vi "Get Key Line.vi"(10 "key description":string, 11 "info data":string) -> (3 "key value":string)   [LabVIEW 2019, in "infolib.lvlib"]
doc: "Remove all sections and returns the rest. Contain infinite loop, but every iteration something should be removed, so the loop should always end."
uses:
  infolib.lvlib
  <vilib>/regexp/Match Regular Expression.xnode
panel:
  # "testing string:"
  # "test1 :: 1\ntest2 :: 22\n#startsection:: 1\nAAA\n#startsection:: 2\nBBB\n\t  \t#endsection:: 2\nCCC\n#endsection:: 1\ntest3::333\n   test4:: 4444\n#startsection:: X\nDDD\n#endsection:: X\ntest5"
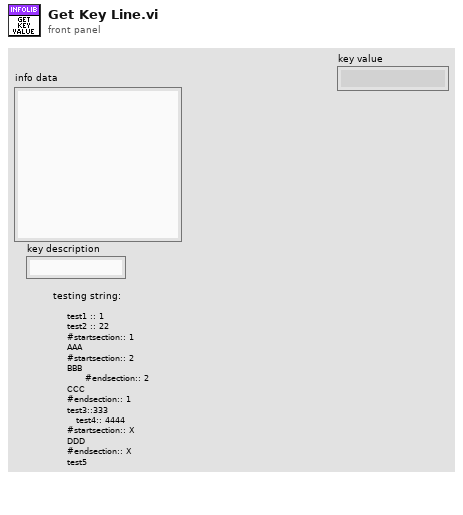
[diagram p1: front panel]
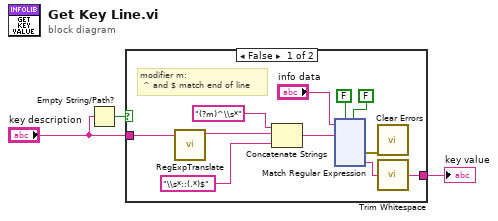
[diagram p0: block diagram]
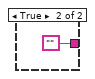
[diagram p2: hidden frame]
diagram:
  n1 = Empty String/Path?(string/path="key description") -> (empty?=w1:bool)
  n2 = case shown="False" w1 {
    tunnel: [w8 ""] -> w3
    tunnel: "key description" -> [w7 _]
    frame False {
      # "modifier m:\n ^ and $ match end of line"
      n3 = call "RegExpTranslate.vi"("string"=w7) -> ("regexp safe string"=w6:string)  [unwired: 10 in]
      n4 = Concatenate Strings("(?m)^\\s*" ("section name"), w6, "\\s*::(.*)$" ("section name")) -> (w9:string)
      n5 = xnode "Match Regular Expression"("input string"="info data", "regular expression"=w9, "ignore case? (F)"=FALSE, "multiline? (F)"=FALSE) -> ("error out"=w13:errorcluster, "submatch 1"=w12:string)  [unwired: 2 in, 4 out]
      n6 = call <vilib>:"Clear Errors.vi"("error in (no error)"=w13) -> ()  [unwired: 5 in, 2 out]
      n7 = call <vilib>:"Trim Whitespace.vi"("string"=w12) -> ("trimmed string"=w8:string)  [unwired: 1 in]
    }
    frame True {
    }
  }
  "key value" <- w3
